vi "ChangeDirection.vi"(8 "error in (no error)":errorcluster, 10 "Direction":T1, 11 "Player in":refnum<class "Player.lvclass">) -> (0 "error out":errorcluster, 3 "Player out":refnum<class "Player.lvclass">)   [LabVIEW 2019, in "Player.lvclass"]
uses:
  Player.lvclass
  Snake/Snake.lvclass
  Direction STYP.ctl
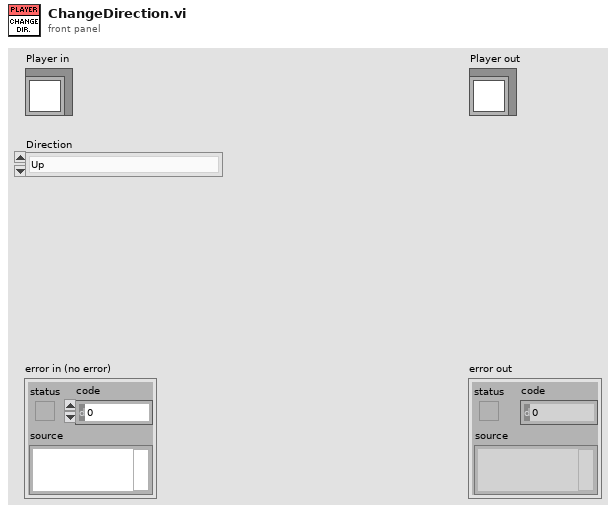
[diagram p1: front panel]
types:
  T1 = typedef "Direction STYP.ctl" = enum16{"Up", "Down", "Left", "Right"}
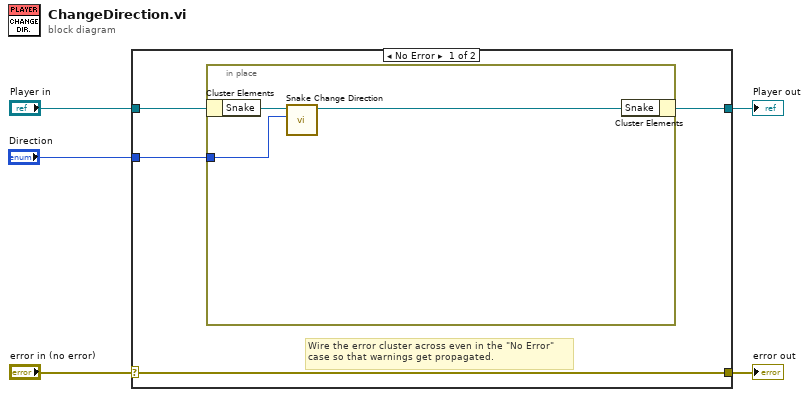
[diagram p0: block diagram]
diagram:
  n1 = case shown="No Error" "error in (no error)" {
    selector: "error in (no error)" -> [w9 w14]
    tunnel: [w9 w14] -> w4
    tunnel: [w8 w13] -> w2
    tunnel: "Player in" -> [w7 w13]
    tunnel: "Direction" -> [w6 _]
    frame No Error {
      # "Wire the error cluster across even in the \"No Error\"\ncase so that warnings get propagated."
      n2 = in-place {
        in-place-border: w6 -> [w10]
        n3 = in-place-cluster #1(w7) -> ("Snake"=w12:refnum<class "Snake.lvclass">)
        n4 = call-dynamic "Snake Change Direction.vi"("Direction"=w10, "Snake in"=w12) -> ("Snake out"=w11:refnum<class "Snake.lvclass">)  [unwired: 8 in, 1 out]
        n5 = in-place-cluster #1("Snake"=w11) -> (w8:refnum<class "Player.lvclass">)
      }
    }
    frame Error {
    }
  }
  "error out" <- w4
  "Player out" <- w2
